vi "DAQ_Fix.vi"(11 "Array in":waveform(dbl)[](array[waveform])) -> (3 "Array out":waveform(dbl)[](array[waveform]))   [LabVIEW 2022 SP3]
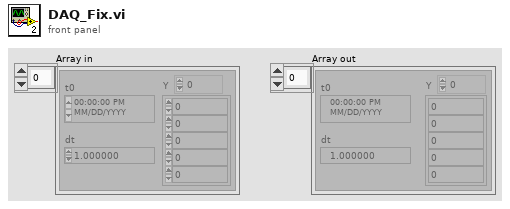
[diagram p1: front panel]
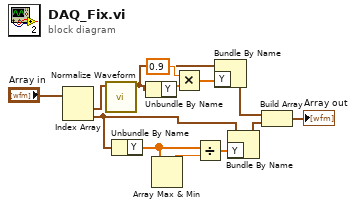
[diagram p0: block diagram]
diagram:
  n1 = Index Array(array="Array in") -> (element #1=w10:waveform(dbl), element #2=w3:waveform(dbl))  [unwired: 2 in]
  n2 = call <vilib>:"Normalize Waveform.vi"("waveform in"=w10) -> ("normalized waveform"=w6:waveform(dbl))  [unwired: 7 in, 3 out]
  n3 = Unbundle By Name(w3) -> ("Y"=w1:dbl[])
  n4 = Unbundle By Name(w6) -> ("Y"=w8:dbl[])
  n5 = Array Max & Min(array=w1) -> (max value=w5:dbl)  [unwired: 3 out]
  n6 = Multiply(x=0.9, y=w8) -> (x*y=w12:dbl[])
  n7 = Divide(x=w1, y=w5) -> (x/y=w4:dbl[])
  n8 = Bundle By Name(cluster=w6, "Y"=w12) -> (w7:waveform(dbl))
  n9 = Bundle By Name(cluster=w3, "Y"=w4) -> (w2:waveform(dbl))
  n10 = Build Array(w7, w2) -> (→"Array out":waveform(dbl)[])
